vi "CAMERATEST.vi"() -> ()   [LabVIEW 2016, in "Test2.lvrbt"]
uses:
  Test2.lvrbt
  <vilib>/NXT/Block Support/NXT_InputPort.ctl
  <vilib>/NXT/Subs/ColorSensorColors.ctl
  <vilib>/NXT/Hardware/Plugins/Tetrix DC Motor/TetrixDCMotorAddress.ctl
  <vilib>/NXT/Hardware/Plugins/Tetrix 180 deg Servo/Tetrix180ServoAddress.ctl
  <vilib>/NXT/NXTIO Xnodes/NXTIONodeSubVIs/TETRIX IO Move Servos.vi
  <vilib>/NXT/Dual Mode Library/Waits/Wait_Num.vi
  <vilib>/NXT/NXTIO Xnodes/NXTIONodeSubVIs/TETRIX IO Move DC Motors.vi
  <vilib>/NXT/Dual Mode Library/Waits/Wait_EV3_Color_Color.vi
  <vilib>/NXT/NXTIO Xnodes/NXTIONodeSubVIs/TETRIX IO Stop DC Motors.vi
  <vilib>/NXT/Dual Mode Library/Sensors/EV3_Ultrasonic_CM.vi
  <vilib>/NXT/NXTIO Xnodes/AddressXNode/NXTIOAddress.xnode
  <vilib>/NXT/Subs/LVHSConnector.ctl
  <vilib>/NXT/NXTIO Xnodes/NXTIOXNode/NXTIO.xnode
  <vilib>/NXT/LegoClasses/BrickReference/BrickReference.lvclass
panel:
  out "Power 2":bool
  out "X Upper Left":u8
  out "X Lower Right":u8
  out "Y Lower Right":u8
  out "Y Upper Left":u8
  out "Count 2":u8
  out "Color 2":u8
  in  "Cluster 2":T1 {"Tracking Mode" items=["Disable Tracking", "Get First Object", "Get n th Object", "Enable Tracking", "Sort Objects  by size", "Sort Objects  by Colors", "Illumination on ", "Illumination Off", "Write Colormap", "Read Colormap", "Line tracking mode", "Object Tracking mode"]}
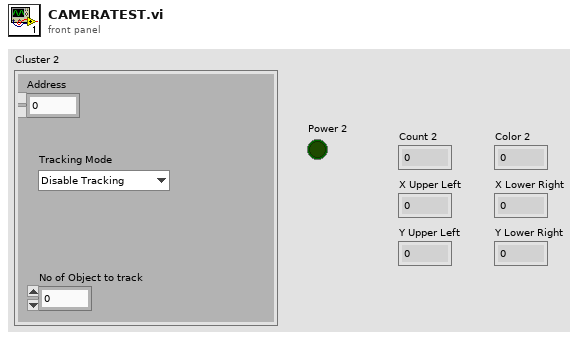
[diagram p1: front panel]
types:
  T1 = cluster{"Address":dbl, "No of Object to track":dbl, "Tracking Mode":u8}
  T2 = typedef "NXT_InputPort.ctl" = u32
  T3 = typedef "ColorSensorColors.ctl" = enum16{"No Color", "Black", "Blue", "Green", "Yellow", "Red", "White", "Brown"}
  T4 = cluster{"Tracking Mode":u8, "Object Number to Track":u8, "Address":u8}
  T5 = typedef "Tetrix180ServoAddress.ctl" = i32
  T6 = cluster{"Tetrix180Servo":T5, "Tetrix180Servo":T5, "Tetrix180Servo":T5, "Tetrix180Servo":T5, "Tetrix180Servo":T5, "Tetrix180Servo":T5}
  T7 = typedef "TetrixDCMotorAddress.ctl" = i32
  T8 = typedef "LVHSConnector.ctl" = refnum<class "BrickReference.lvclass">
  T9 = cluster{"TetrixDCMotor":T7, "TetrixDCMotor 2":T7}
  T10 = cluster{"Total Tracked Objects":u8, "Color":u8, "X Upper Left":u8, "Y Upper Left":u8, "X Lower Right":u8, "Y Lower Right":u8, "Status (boolean)":bool}
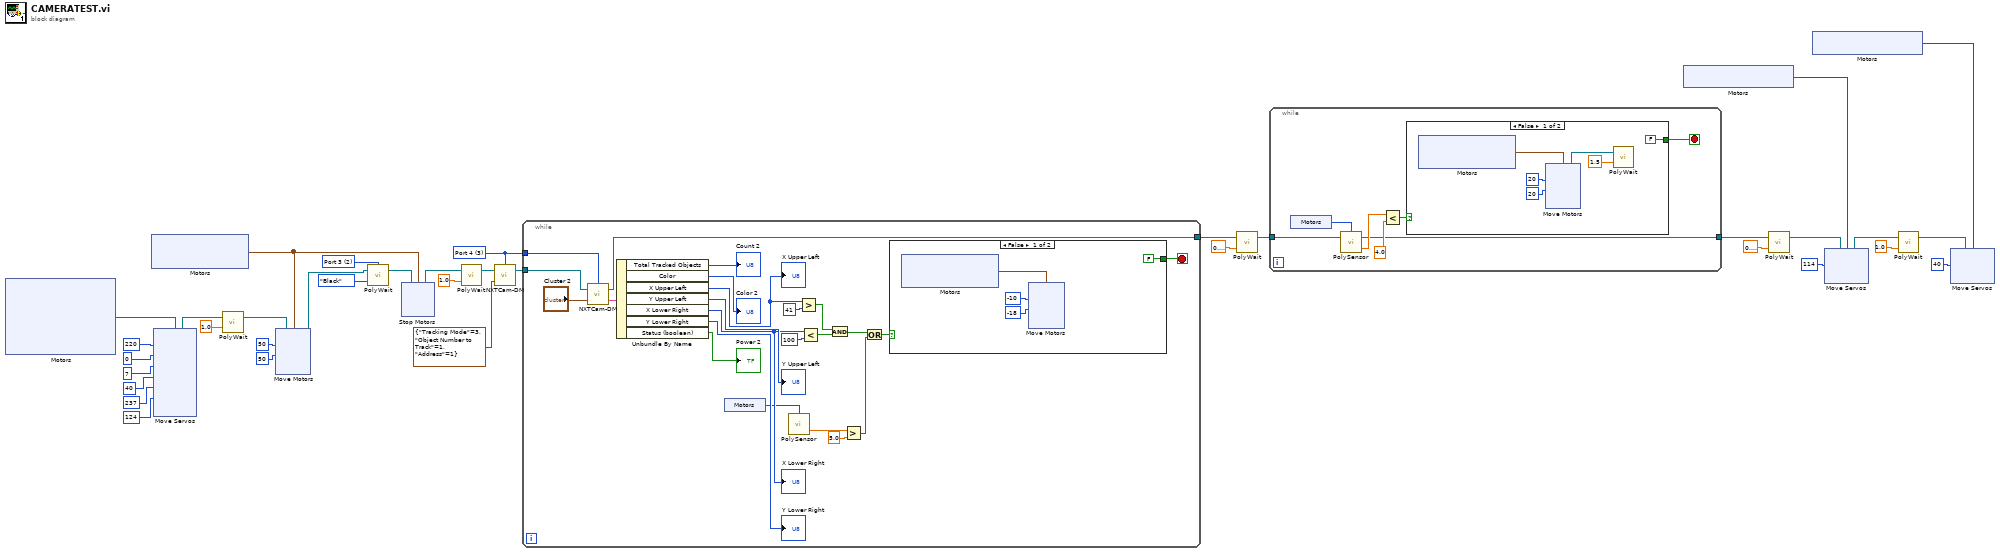
[diagram p0: block diagram]
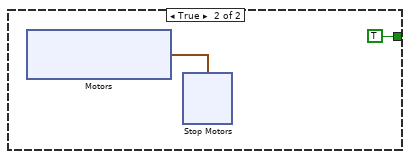
[diagram p2: hidden frame]
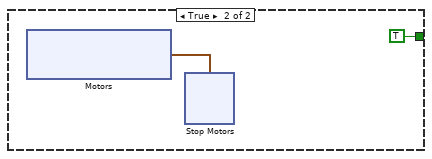
[diagram p3: hidden frame]
diagram:
  w16 = T2 2 items=["Port 1", "Port 2", "Port 3", "Port 4"] ("Port (Port 1)")
  w14 = T2 3 items=["Port 1", "Port 2", "Port 3", "Port 4"] ("Input Port")
  n1 = xnode "Motors"() -> ("Motor"=w29:T6)
  n2 = xnode "Motors"() -> ("Motor"=w33:cluster{"TetrixDCMotor":T7, "TetrixDCMotor":T7})
  n3 = xnode "Move Servos"("Position 6"=u8 124, "Position 5"=u8 237, "Position 4"=u8 40, "Position 3"=u8 7, "Position 2"=u8 0, "Position 1"=u8 220, "Motors"=w29) -> ("NXT/EV3"=w21:T8)  [unwired: 1 in]
  n4 = call-poly <vilib>:"PolyWait.vi"("Time (1 sec)"=sgl 1.0, "NXT/EV3"=w21) -> ("NXT/EV3"=w17:T8)  [unwired: 2 in]
  n5 = xnode "Move Motors"("Power/Speed 2"=i8 50, "Power/Speed 1"=i8 50, "Motors"=w33, "NXT/EV3"=w17) -> ("NXT/EV3"=w19:T8)
  n6 = call-poly <vilib>:"PolyWait.vi"("Color (Red)"=ColorSensorColors."Black", "NXT/EV3"=w19, "Port (Port 1)"=w16) -> ("NXT/EV3"=w18:T8)  [unwired: 1 in]
  n7 = xnode "Stop Motors"("Motors"=w33, "NXT/EV3"=w18) -> ("NXT/EV3"=w32:T8)
  n8 = call-poly <vilib>:"PolyWait.vi"("Time (1 sec)"=sgl 1.0, "NXT/EV3"=w32) -> ("NXT/EV3"=w31:T8)  [unwired: 2 in]
  n9 = call "NXTCam-DM.vi"("Input of NXTCam"=T4 {"Tracking Mode"=3, "Object Number to Track"=1, "Address"=1}, "NXT"=w31, "Input Port"=w14) -> ("NXT dup"=w15:T8)  [unwired: 1 out]
  n10 = while {
    tunnel: w15 -> [w47]
    tunnel: w14 -> [w46]
    tunnel: [w44] -> w12
    stop <- w45 stop-if-true
    n11 = call "NXTCam-DM.vi"("Input of NXTCam"="Cluster 2", "NXT"=w47, "Input Port"=w46) -> ("Output of NXTCam"=w54:T10, "NXT dup"=w44:T8)
    n12 = Unbundle By Name(w54) -> ("Total Tracked Objects"=→"Count 2":u8, "Color"=→"Color 2":u8, "X Upper Left"=w43:u8, "Y Upper Left"=→"Y Upper Left":u8, "X Lower Right"=w51:u8, "Y Lower Right"=→"Y Lower Right":u8, "Status (boolean)"=→"Power 2":bool)
    "X Upper Left" <- w43
    "X Lower Right" <- w51
    n13 = xnode "Motors"() -> ("Sensor"=w37:T2)
    n14 = call-poly <vilib>:"PolySensor.vi"("Port (Port 1)"=w37) -> ("Centimeters"=w39:sgl)  [unwired: 2 in, 1 out]
    n15 = Greater?(x=w43, y=u8 41) -> (0:w49:bool)
    n16 = Less?(x=w51, y=u8 100) -> (x < y?=w48:bool)
    n17 = And(x=w49, y=w48) -> (x .and. y?=w41:bool)
    n18 = Greater?(x=w39, y=sgl 5.0) -> (0:w38:bool)
    n19 = Or(x=w41, y=w38) -> (x .or. y?=w40:bool)
    n20 = case shown="False" w40 {
      tunnel: [FALSE TRUE] -> w45
      frame False {
        n21 = xnode "Motors"() -> ("Motor"=w64:cluster{"TetrixDCMotor":T7, "TetrixDCMotor":T7})
        n22 = xnode "Move Motors"("Power/Speed 2"=i8 -18, "Power/Speed 1"=i8 -10, "Motors"=w64) -> ()  [unwired: 1 in, 1 out]
      }
      frame True {
        n23 = xnode "Motors"() -> ("Motor"=w75:cluster{"TetrixDCMotor":T7, "TetrixDCMotor":T7})
        n24 = xnode "Stop Motors"("Motors"=w75) -> ()  [unwired: 1 in, 1 out]
      }
    }
  }
  n25 = call-poly <vilib>:"PolyWait.vi"("Time (1 sec)"=sgl 0.8, "NXT/EV3"=w12) -> ("NXT/EV3"=w11:T8)  [unwired: 2 in]
  n26 = while {
    tunnel: w11 -> [w88]
    tunnel: [w83] -> w9
    stop <- w85 stop-if-true
    n27 = xnode "Motors"() -> ("Sensor"=w82:T2)
    n28 = call-poly <vilib>:"PolySensor.vi"("NXT/EV3"=w88, "Port (Port 1)"=w82) -> ("Centimeters"=w87:sgl, "NXT/EV3"=w83:T8)  [unwired: 1 in]
    n29 = Less?(x=w87, y=sgl 4.0) -> (x < y?=w84:bool)
    n30 = case shown="False" w84 {
      tunnel: [FALSE TRUE] -> w85
      frame False {
        n31 = xnode "Motors"() -> ("Motor"=w95:cluster{"TetrixDCMotor":T7, "TetrixDCMotor":T7})
        n32 = xnode "Move Motors"("Power/Speed 2"=i8 20, "Power/Speed 1"=i8 20, "Motors"=w95) -> ("NXT/EV3"=w92:T8)  [unwired: 1 in]
        n33 = call-poly <vilib>:"PolyWait.vi"("Time (1 sec)"=sgl 1.5, "NXT/EV3"=w92) -> ()  [unwired: 2 in, 1 out]
      }
      frame True {
        n34 = xnode "Motors"() -> ("Motor"=w106:cluster{"TetrixDCMotor":T7, "TetrixDCMotor":T7})
        n35 = xnode "Stop Motors"("Motors"=w106) -> ()  [unwired: 1 in, 1 out]
      }
    }
  }
  n36 = xnode "Motors"() -> ("Motor"=w7:T5)
  n37 = call-poly <vilib>:"PolyWait.vi"("Time (1 sec)"=sgl 0.8, "NXT/EV3"=w9) -> ("NXT/EV3"=w8:T8)  [unwired: 2 in]
  n38 = xnode "Motors"() -> ("Motor"=w3:T5)
  n39 = xnode "Move Servos"("Position 1"=u8 114, "Motors"=w7, "NXT/EV3"=w8) -> ("NXT/EV3"=w5:T8)
  n40 = call-poly <vilib>:"PolyWait.vi"("Time (1 sec)"=sgl 1.0, "NXT/EV3"=w5) -> ("NXT/EV3"=w1:T8)  [unwired: 2 in]
  n41 = xnode "Move Servos"("Position 1"=u8 40, "Motors"=w3, "NXT/EV3"=w1) -> ()  [unwired: 1 out]
